vi "SCPI_sending_reading_V2.vi"(4 "error in (no error)":errorcluster, 5 "Numeric entrece":dbl, 6 "SCIPI":T1 items=["*IDN?", "*SAV 1", "*RCL 1", "INSTTrument CH1", "INSTTrument CH2", "INSTrument?", "MEASure:CURRent? CH1", "MEASure:CURRent? CH2", "MEASure:VOLTage? CH1", "MEASure:VOLTage? CH2", "MEASure:POWEr? CH1", "MEASure:POWEr? CH2", "CH1:CURRent?", "CH2:CURRent?", "CH1:VOLTage? ", "CH2:VOLTage? ", "OUTPut CH1,ON", "OUTPut CH1,OFF", "OUTPut CH2,ON", "OUTPut CH2,OFF", "OUTPut CH3,ON", "OUTPut CH3,OFF", "OUTPut:TRACK 0", "OUTPut:TRACK 1", "OUTPut:TRACK 2", "OUTPut:WAVE CH1,ON", "OUTPut:WAVE CH1,OFF", "OUTPut:WAVE CH2,ON", "OUTPut:WAVE CH2,OFF"], 7 "VISA":refnum<visa-resource-name>) -> (0 "error out":errorcluster, 1 "read numeric value":dbl, 2 "read buffer - string":string, 3 "VISA resource name out":refnum<visa-resource-name>)   [LabVIEW 2020]
doc: "Wysyłanie podstawowych komend SCPI - zasilacz SIGLENT SPD3303X-E"
uses:
  controls/SCPI_enum.ctl
panel:
  in  "byte count":u32=4096
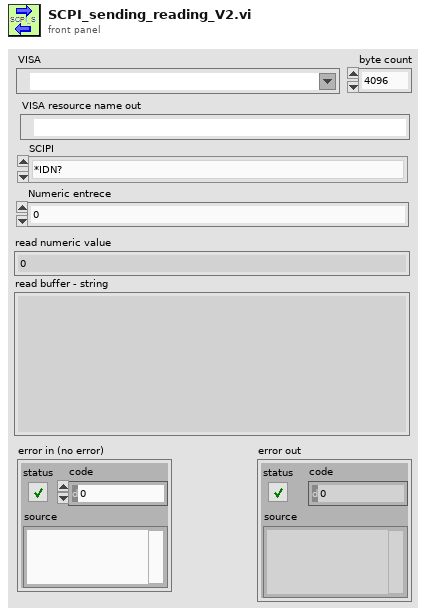
[diagram p1: front panel]
types:
  T1 = typedef "SCPI_enum.ctl" = u16
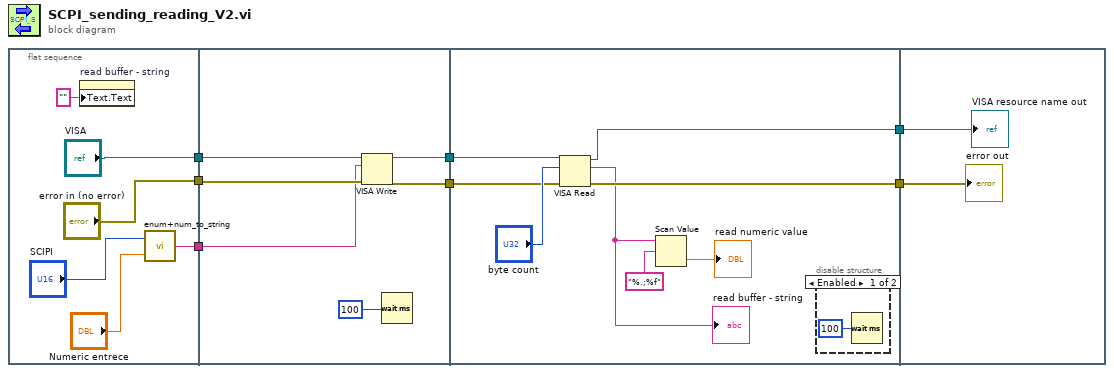
[diagram p0: block diagram]
diagram:
  n1 = flat-sequence {
    tunnel: ["VISA"] -> w7
    tunnel: ["error in (no error)"] -> w3
    tunnel: [w9] -> w1
    tunnel: w7 -> [w18]
    tunnel: [w17] -> w5
    tunnel: [w16] -> w4
    tunnel: w3 -> [w15]
    tunnel: w1 -> [w14]
    tunnel: [w26] -> w6
    tunnel: w5 -> [w25]
    tunnel: w4 -> [w24]
    tunnel: [w23] -> w2
    tunnel: w6 -> [w30]
    tunnel: w2 -> [w29]
    frame #0 {
      n2 = property on="read buffer - string" class="Str"("Text.Text"="") -> ()  [unwired: 2 in, 2 out]
      n3 = call "enum+num_to_string.vi"("Numeric"="Numeric entrece", "SCIPI"="SCIPI") -> ("concatenated string"=w9:string)
    }
    frame #1 {
      n4 = VISA Write(VISA resource name=w18, write buffer=w14, error in (no error)=w15) -> (VISA resource name out=w17:refnum<visa-resource-name>, error out=w16:errorcluster)  [unwired: 1 out]
      n5 = Wait (ms)(milliseconds to wait=u32 100) -> ()  [unwired: 1 out]
    }
    frame #2 {
      n6 = VISA Read(VISA resource name=w25, byte count="byte count", error in (no error)=w24) -> (VISA resource name out=w23:refnum<visa-resource-name>, read buffer=w20:string, error out=w26:errorcluster)  [unwired: 1 out]
      "read buffer - string" <- w20
      n7 = Scan Value(string=w20, format string="%.;%f") -> (value=→"read numeric value":dbl)  [unwired: 1 in, 1 out]
      n8 = disable-structure shown="Enabled" {
        frame Enabled {
          n9 = Wait (ms)(milliseconds to wait=u32 100) -> ()  [unwired: 1 out]
        }
        frame Disabled {
        }
      }
    }
    frame #3 {
      "error out" <- w30
      "VISA resource name out" <- w29
    }
  }
